vi "Calculate Lineout and Centroid.vi"(8 "error in (no error)":errorcluster, 10 "Lineout IN":T4, 11 "Image":T3) -> (0 "error out":errorcluster, 2 "Histogram OUT":T1, 3 "Lineout Out":T2)   [LabVIEW 2020]
doc: "Calculates lineout and cetriod\ninput\n1. image\n2. input cluster\n\noutput\n1. image out\n2. output cluster(lineout and centriod cluster)"
uses:
  <vilib>/vision/Image Controls.llb/IMAQ Image.ctl
  <vilib>/vision/NI_Vision_Development_Module.lvlib
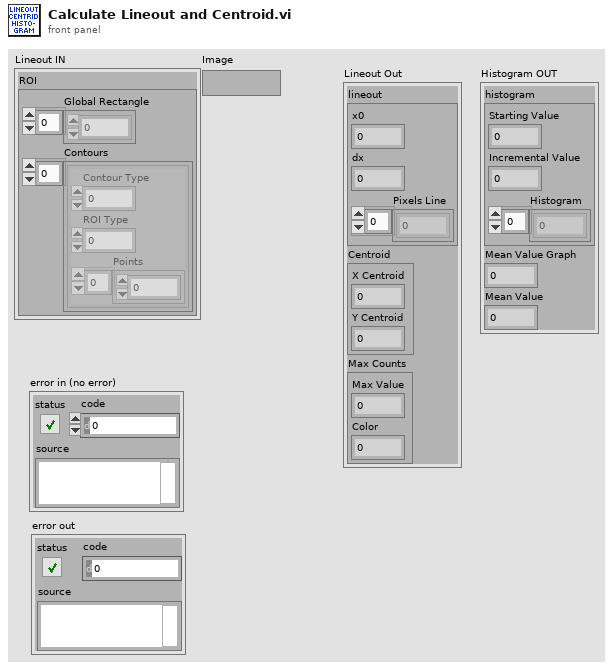
[diagram p1: front panel]
types:
  T1 = cluster{"histogram":cluster{"Starting Value":sgl, "Incremental Value":sgl, "Histogram":u32[]}, "Mean Value Graph":sgl, "Mean Value":sgl}
  T2 = cluster{"lineout":cluster{"x0":sgl, "dx":sgl, "Pixels Line":sgl[]}, "Centroid":cluster{"X Centroid":sgl, "Y Centroid":sgl}, "Max Counts":cluster{"Max Value":sgl, "Color":u32}}
  T3 = typedef "IMAQ Image.ctl" = refnum<image>
  T4 = cluster{"ROI":cluster{"Global Rectangle":i32[], "Contours":cluster{"Contour Type":u32, "ROI Type":u32, "Points":i32[]}[]}}
  T5 = cluster{"Global Rectangle":i32[], "Contours":cluster{"Contour Type":u32, "ROI Type":u32, "Points":i32[]}[]}
  T6 = typedef "IMAQ Line" = cluster{"Start X":i32, "Start Y":i32, "End X":i32, "End Y":i32}
  T7 = cluster{"Starting Value":sgl, "Incremental Value":sgl, "Histogram":u32[]}
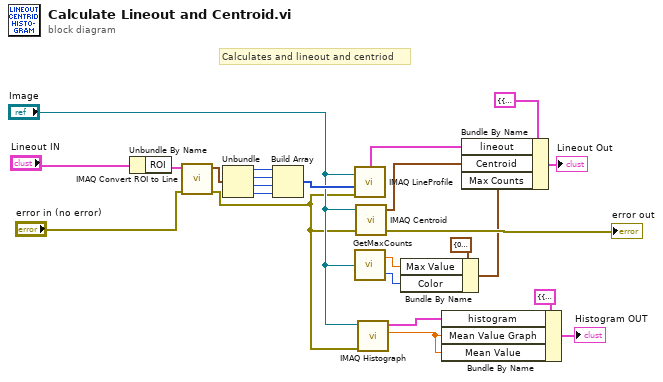
[diagram p0: block diagram]
diagram:
  # "Calculates and lineout and centriod"
  n1 = Unbundle By Name("Lineout IN") -> ("ROI"=w21:T5)
  n2 = call "IMAQ Convert ROI to Line"("error in (no error)"="error in (no error)", "ROI Descriptor"=w21) -> ("error out"=w1:errorcluster, "Line"=w19:T6)  [unwired: 7 in]
  n3 = Unbundle(w19) -> ("Start X"=w15:i32, "Start Y"=w16:i32, "End X"=w17:i32, "End Y"=w18:i32)
  n4 = Build Array(w15, w16, w17, w18) -> (w20:i32[])
  n5 = call "IMAQ LineProfile"("error in (no error)"=w1, "Line Coordinates"=w20, "Image"="Image") -> ("Line Graph"=w22:cluster{"x0":sgl, "dx":sgl, "Pixels Line":sgl[]})  [unwired: 2 in, 3 out]
  n6 = call "GetMaxCounts.vi"("New Image"="Image") -> ("Maximal Value"=w10:sgl, "Color"=w9:u32)
  n7 = call "IMAQ Centroid"("error in (no error)"=w1, "Image"="Image") -> ("error out"=→"error out":errorcluster, "Centroid"=w23:cluster{"X Centroid":sgl, "Y Centroid":sgl})  [unwired: 2 in]
  n8 = call "IMAQ Histograph"("error in (no error)"=w1, "Image"="Image") -> ("Mean Value"=w3:sgl, "Histogram Graph"=w4:T7)  [unwired: 6 in, 2 out]
  n9 = Bundle By Name(cluster=cluster{"Max Value":sgl, "Color":u32} {"Max Value"=0.0, "Color"=0} ("Max Counts"), "Max Value"=w10, "Color"=w9) -> (w8:cluster{"Max Value":sgl, "Color":u32})
  n10 = Bundle By Name(cluster=T1 {"histogram"={"Starting Value"=0.0, "Incremental Value"=0.0, "Histogram"=[]}, "Mean Value Graph"=0.0, "Mean Value"=0.0} ("Histogram OUT"), "histogram"=w4, "Mean Value Graph"=w3, "Mean Value"=w3) -> (→"Histogram OUT":T1)
  n11 = Bundle By Name(cluster=T2 {"lineout"={"x0"=0.0, "dx"=0.0, "Pixels Line"=[]}, "Centroid"={"X Centroid"=0.0, "Y Centroid"=0.0}, "Max Counts"={"Max Value"=0.0, "Color"=0}} ("Lineout Out"), "lineout"=w22, "Centroid"=w23, "Max Counts"=w8) -> (→"Lineout Out":T2)
